vi "set control visibility.vi"(2 "error in":errorcluster, 3 "Disabled":T1(ring), 4 "Controls Reference Array":refnum<vi>[](array[refnum])) -> (0 "error out":errorcluster)   [LabVIEW 2020]
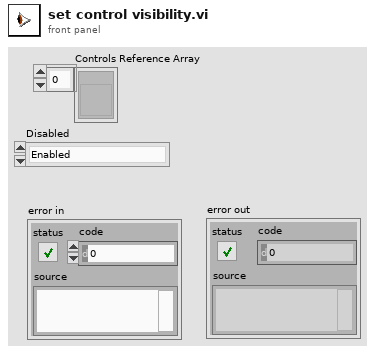
[diagram p1: front panel]
types:
  T1 = enum8{"Enabled", "Disabled", "Disabled and Grayed Out"}
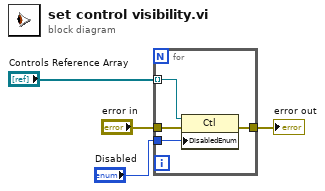
[diagram p0: block diagram]
diagram:
  n1 = for {
    tunnel: "Disabled" -> [w8]
    tunnel: "error in" -> [w7]
    tunnel: [w6] -> w2
    tunnel: "Controls Reference Array" -> [w5] mode=indexing
    n2 = property on="Property Node" class="Ctl"(reference=w5, error in=w7, "DisabledEnum"=w8) -> (error out=w6:errorcluster)  [unwired: 1 out]
  }
  "error out" <- w2
